vi "Disconnect.vi"(8 "error in (no error)":errorcluster, 11 "PQ Connection in":refnum<class "PQ Connection.lvclass">) -> (0 "error out":errorcluster)   [LabVIEW 2015, in "PQ Connection.lvclass"]
doc: "Disconnects from teh PostgreSQL database. This operates even if there is an error in."
uses:
  PQ Connection.lvclass
  PQ Connection.lvclass/PQ Connection.ctl
  libpq.dll
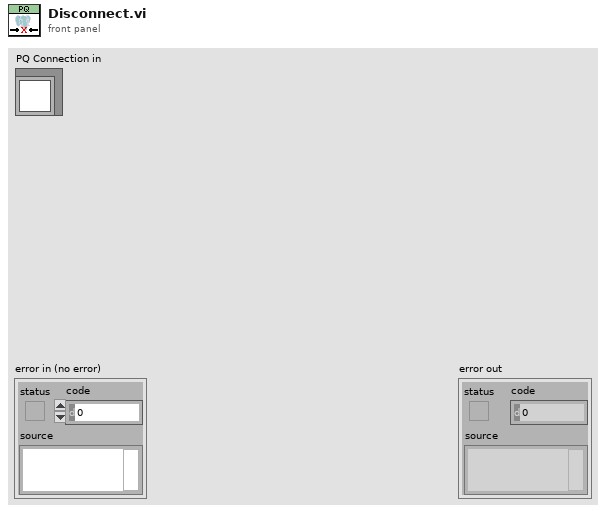
[diagram p1: front panel]
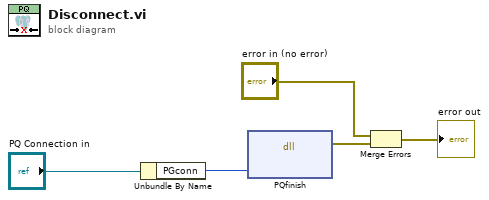
[diagram p0: block diagram]
diagram:
  n1 = Unbundle By Name("PQ Connection in") -> ("PGconn"=w3:u32)
  n2 = dll-call lib="C:/PQ/Connection/libpq.dll" fn="PQfinish"("PGconn"=w3) -> (error out=w1:errorcluster)  [unwired: 5 in, 1 out]
  n3 = Merge Errors("error in (no error)", w1) -> (→"error out":errorcluster)
